vi "GetAllTempSaveNames.vi"(1 "String":string) -> (0 "Array":string[](array[string]))   [LabVIEW 2014]
uses:
  TempConfig.ctl
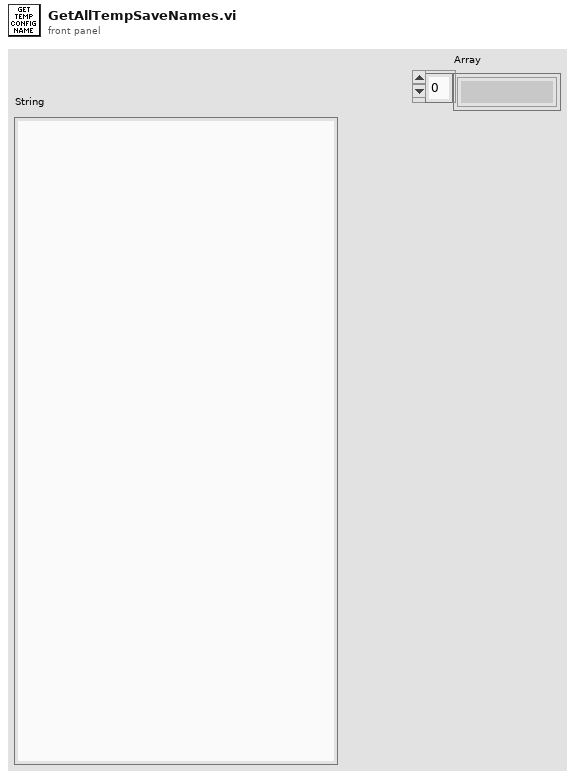
[diagram p1: front panel]
types:
  T1 = typedef "TempConfig.ctl" = cluster{"Name":string, "Thi":dbl, "Tlow":dbl, "Tstartup":dbl, "P":dbl, "I":dbl, "D":dbl, "Ilim":dbl, "Vlim":dbl, "Default":bool}
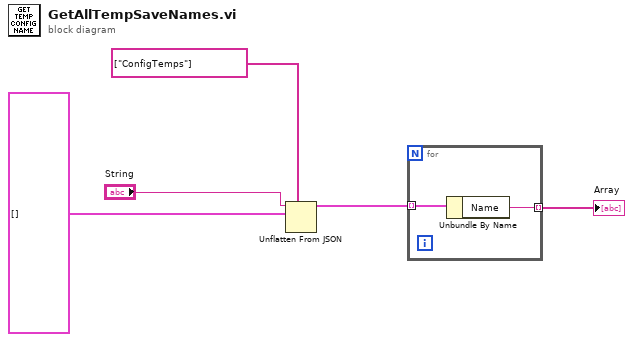
[diagram p0: block diagram]
diagram:
  n1 = Unflatten From JSON(path=string[] ["ConfigTemps"], JSON string="String", type and defaults=T1[] []) -> (value=w3:T1[])  [unwired: 4 in, 1 out]
  n2 = for {
    tunnel: w3 -> [w7] mode=indexing
    tunnel: [w6] -> w1 mode=indexing
    n3 = Unbundle By Name(w7) -> ("Name"=w6:string)
  }
  "Array" <- w1
